vi "CheckBaxterEnabled.vi"(0 "error in":errorcluster, 3 "node":string) -> (1 "error out":errorcluster)   [LabVIEW 2012]
doc: "Enables motors, calibrates grippers"
uses:
  <userlib>/ROSforLV/ROS/Code/SubVIs/BaxterSide.ctl
panel:
  in  "Nodes Enabled":string[](array[string])
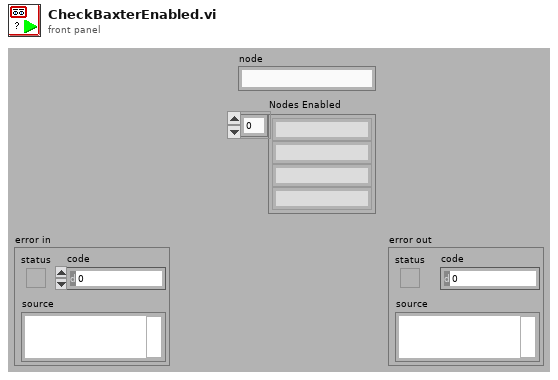
[diagram p1: front panel]
types:
  T1 = typedef "BaxterSide.ctl" = enum16{"left", "right"}
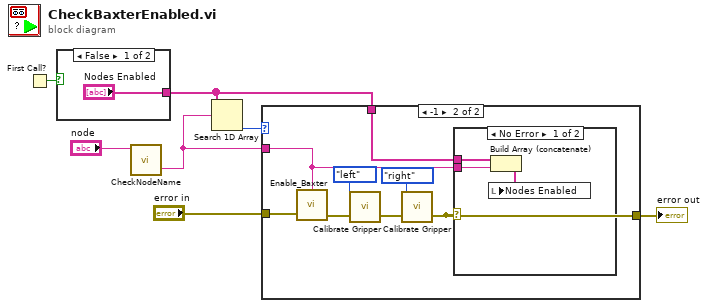
[diagram p0: block diagram]
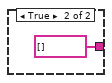
[diagram p2: hidden frame]
diagram:
  n1 = First Call?() -> (First Call?: T/F=w1:bool)
  n2 = case shown="False" w1 {
    tunnel: ["Nodes Enabled" string[] [] ("Nodes Enabled")] -> w4
    frame False {
    }
    frame True {
    }
  }
  n3 = call <userlib>:"CheckNodeName.vi"("node"="node") -> ("name"=w2:string)  [unwired: 1 in, 1 out]
  n4 = Search 1D Array(1D array=w4, element=w2) -> (index of element=w5:i32)  [unwired: 1 in]
  n5 = case shown="-1" w5 {
    tunnel: "error in" -> [w10 w14]
    tunnel: [w10 w13] -> w6
    tunnel: w2 -> [_ w11]
    tunnel: w4 -> [_ w12]
    frame Default {
    }
    frame -1 {
      n6 = call <userlib>:"Enable_Baxter.vi"("error in"=w14, "node"=w11) -> ("error out"=w18:errorcluster)  [unwired: 2 in]
      n7 = call <userlib>:"Calibrate Gripper.vi"("Side"=BaxterSide."left", "error in"=w18) -> ("error out"=w16:errorcluster)  [unwired: 4 in]
      n8 = call <userlib>:"Calibrate Gripper.vi"("Side"=BaxterSide."right", "error in"=w16) -> ("error out"=w13:errorcluster)  [unwired: 4 in]
      n9 = case shown="No Error" w13 {
        tunnel: w12 -> [w21 _]
        tunnel: w11 -> [w20 _]
        frame No Error {
          n10 = Build Array (concatenate)(w21, w20) -> (w19:string[])
          n11 = local write "Nodes Enabled"(w19) -> ()
        }
        frame Error {
        }
      }
    }
  }
  "error out" <- w6
